vi "Wheel_coupled (SubVI).vi"(8 "Error In":errorcluster, 11 "LINX Resource":T1) -> (0 "error out":errorcluster, 3 "Speed plot":dbl(graph))   [LabVIEW 2020]
uses:
  <vilib>/MakerHub/LINX/Private/Type Defs/LINX Ref.ctl
  <vilib>/MakerHub/LINX/Private/Type Defs/Platform.ctl
  <vilib>/MakerHub/LINX/Private/Type Defs/Interface.ctl
  <vilib>/MakerHub/LINX/Private/Device/Type Defs/LINX Device Config.ctl
  <vilib>/MakerHub/LINX/Private/Device/Type Defs/TCP Config.ctl
  <vilib>/MakerHub/LINX/Private/Device/Type Defs/Channels.ctl
  <vilib>/MakerHub/LINX/Public/Peripherals/Digital/Digital Write 1 Chan.vi
  <vilib>/MakerHub/LINX/Public/Peripherals/Digital/Digital Write N Chans.vi
  <vilib>/MakerHub/LINX/Private/Local IO/LinxDigitalWrite.vi
  <vilib>/MakerHub/LINX/Public/Utilities/Check Channel.vi
  Shared/ModuleCrosstalk/Crosstalk.vi
  <vilib>/MakerHub/LINX/Private/Utilties/Generate Error.vi
  <vilib>/MakerHub/LINX/LMH-LINX.lvlib
  <vilib>/MakerHub/LINX/Private/Device/Device.lvlib
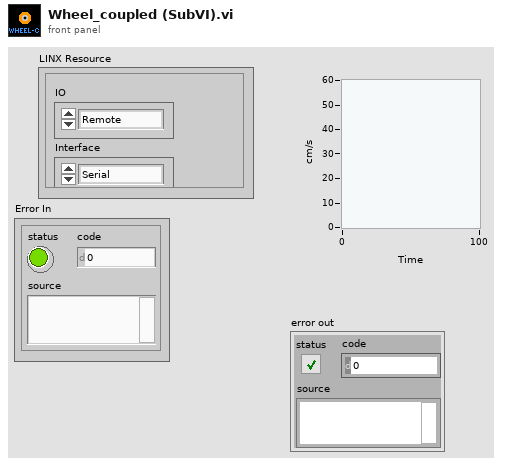
[diagram p1: front panel]
types:
  T1 = typedef "LMH-LINX.lvlib/LINX Ref.ctl" = cluster{"IO":T2, "Interface":T3, "LINX Device Config":T4}
  T2 = typedef "LMH-LINX.lvlib/Platform.ctl" = enum16{"Remote", "Local"}
  T3 = typedef "LMH-LINX.lvlib/Interface.ctl" = enum16{"Serial", "TCP"}
  T4 = typedef "LMH-LINX.lvlib/Device.lvlib/LINX Device Config.ctl" = cluster{"Interface":T3, "COM Port":refnum<visa-resource-name>, "TCP Configuration":T5, "Device Family":u8, "Device ID":u8, "Device Name":string, "TCP Ref":refnum<k5>, "Channels":T6}
  T5 = typedef "LMH-LINX.lvlib/Device.lvlib/TCP Config.ctl" = cluster{"IP Address":string, "Port":u16}
  T6 = typedef "LMH-LINX.lvlib/Channels.ctl" = cluster{"DI":u8[], "DO":u8[], "AI":u8[], "AO":u8[], "PWM":u8[], "QE":u8[], "UART":u8[], "I2C 2":u8[], "SPI":u8[], "CAN":u8[], "Servo":u8[], "AI Ref (V)":dbl, "AI Resolution (Bits)":u8, "AO Ref (V)":dbl, "AO Resolution (Bits)":u8}
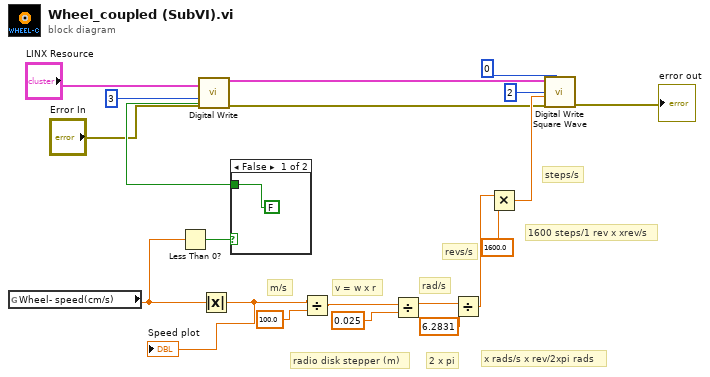
[diagram p0: block diagram]
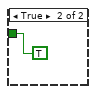
[diagram p2: hidden frame]
diagram:
  # "steps/s"
  # "1600 steps/1 rev x xrev/s"
  # "x rads/s x rev/2xpi rads"
  # "2 x pi"
  # "revs/s"
  # "rad/s"
  # "radio disk stepper (m)"
  # "v = w x r"
  # "m/s"
  n1 = global read "Crosstalk.vi" "Wheel- speed(cm/s)"() -> (w17:dbl)
  n2 = Less Than 0?(x=w17) -> (x < 0?=w9:bool)
  n3 = Absolute Value(x=w17) -> (abs(x)=w20:dbl)
  "Speed plot" <- w20
  n4 = case shown="False" w9 {
    tunnel: [FALSE ("Output Value") TRUE ("Output Value")] -> w10
    frame False {
    }
    frame True {
    }
  }
  n5 = call-poly <vilib>:"Digital Write.vi"("Error In"="Error In", "Output Value"=w10, "DO Channel"=u8 3, "LINX Resource"="LINX Resource") -> ("Error Out"=w5:errorcluster, "LINX Resource"=w4:T1)  [unwired: 6 in]
  n6 = Divide(x=w20, y=100.0 ("Frequency (Hz)")) -> (x/y=w19:dbl)
  n7 = Divide(x=w19, y=0.025) -> (x/y=w12:dbl)
  n8 = Divide(x=w12, y=6.2831) -> (x/y=w14:dbl)
  n9 = Multiply(x=w14, y=1600.0) -> (x*y=w16:dbl)
  n10 = call <vilib>:"Digital Write Square Wave.vi"("Duration (ms)"=u32 0, "Error In"=w5, "Frequency (Hz)"=w16, "Channel"=u8 2, "LINX Resource"=w4) -> ("Error Out"=→"error out":errorcluster)  [unwired: 5 in, 1 out]
